vi "Close (System).vi"(8 "error in (no error)":errorcluster, 11 "Session in":refnum<k21>="localhost") -> (0 "error out":errorcluster)   [LabVIEW 2012, in "nisyscfg.lvlib"]
doc: "Closes a reference to a system."
uses:
  <vilib>/nisyscfg/nisyscfg.lvlib
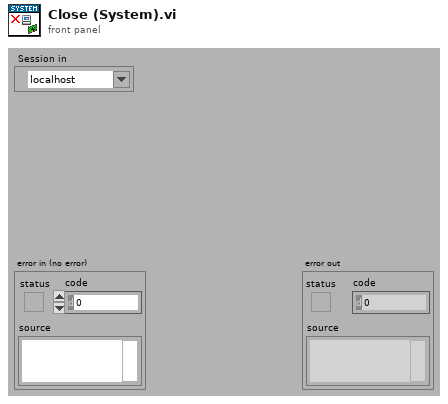
[diagram p1: front panel]
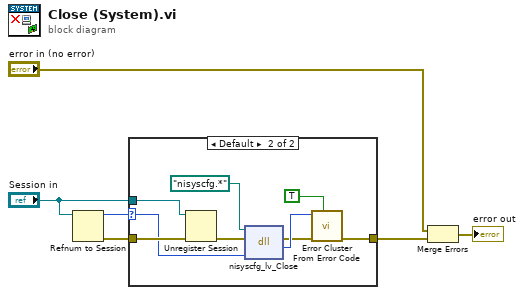
[diagram p0: block diagram]
diagram:
  n1 = Refnum to Session(7:"Session in") -> (0:w2:errorcluster, 3:w1:u64)  [unwired: 1 in]
  n2 = case shown="Default" w1 {
    selector: w1 -> [_ w8]
    tunnel: "Session in" -> [_ w16]
    tunnel: [w7 w15] -> w3
    tunnel: w2 -> [w7 w9]
    frame 0 {
      # "Unlike refnums, closing an I/O control\nthat has not been opened, or is closed\ntwice, is not an error."
    }
    frame Default {
      n3 = Unregister Session(8:w9, 11:w16) -> (0:w10:errorcluster)
      n4 = dll-call lib="nisyscfg.*" fn="nisyscfg_lv_Close" label="Close"(path in=path "nisyscfg.*", error in=w10, "framework"=w8) -> (error out=w13:errorcluster, "status"=w14:i32)  [unwired: 1 in, 2 out]
      n5 = call <vilib>:"Error Cluster From Error Code.vi"("show call chain? (False)"=TRUE, "error in (no error)"=w13, "error code (0)"=w14) -> ("error out"=w15:errorcluster)  [unwired: 6 out]
    }
  }
  n6 = Merge Errors("error in (no error)", w3) -> (→"error out":errorcluster)
